vi "VT100Codes.vi"(10 "read buffer":string="\u001b[0m\u001b[01;34mmicropython-serial-0.3\u001b[0m         \u001b[01;34mrequests-2.22.0\u001b[0m\n\u001b[01;31mmicropython-serial-0.3.tar.gz\u001b[0m  \u001b[01;31mrequests-2.22.0.tar.gz\u001b[0m\nrobot@ev3dev:~$ ", 11 "Console In":string="\r\n\r\nLinux ev3dev 4.14.117-ev3dev-2.3.4-ev3 #1 PREEMPT Thu May 9 15:13:01 CDT 2019 armv5tejl\r\n             _____     _\r\n   _____   _|___ /  __| | _____   __\r\n  / _ \\ \\ / / |_ \\ / _` |/ _ \\ \\ / /\r\n |  __/\\ V / ___) | (_| |  __/\\ V /\r\n  \\___| \\_/ |____/ \\__,_|\\___| \\_/\r\n\r\nDebian stretch on LEGO MINDSTORMS EV3!\r\nLast login: Thu Feb 13 18:25:48 2020 from 130.64.189.217\r\r\nrobot@ev3dev:~$ \r\nrobot@ev3dev:~$ \r\nrobot@ev3dev:~$ brickrun -r --  pybricks-micropython\r\nPybricks MicroPython fc828f94 on 2020-01-30; linux version\r\nUse Ctrl-D to exit, Ctrl-E for paste mode\r\n>>> \nrobot@ev3dev:~$ ls\n") -> (3 "Console Out":string="\r\n\r\nLinux ev3dev 4.14.117-ev3dev-2.3.4-ev3 #1 PREEMPT Thu May 9 15:13:01 CDT 2019 armv5tejl\r\n             _____     _\r\n   _____   _|___ /  __| | _____   __\r\n  / _ \\ \\ / / |_ \\ / _` |/ _ \\ \\ / /\r\n |  __/\\ V / ___) | (_| |  __/\\ V /\r\n  \\___| \\_/ |____/ \\__,_|\\___| \\_/\r\n\r\nDebian stretch on LEGO MINDSTORMS EV3!\r\nLast login: Thu Feb 13 18:25:48 2020 from 130.64.189.217\r\r\nrobot@ev3dev:~$ \r\nrobot@ev3dev:~$ \r\nrobot@ev3dev:~$ brickrun -r --  pybricks-micropython\r\nPybricks MicroPython fc828f94 on 2020-01-30; linux version\r\nUse Ctrl-D to exit, Ctrl-E for paste mode\r\n>>> ")   [LabVIEW 2020]
uses:
  ColorText/ColorGlobals.vi
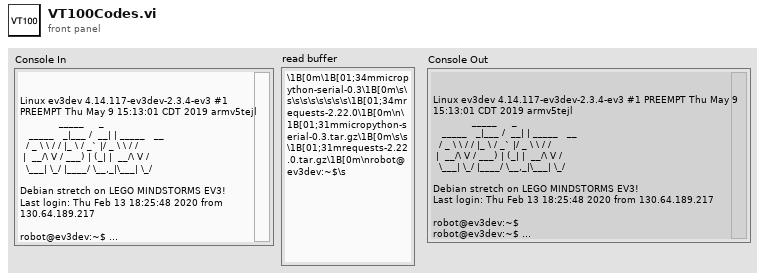
[diagram p1: front panel]
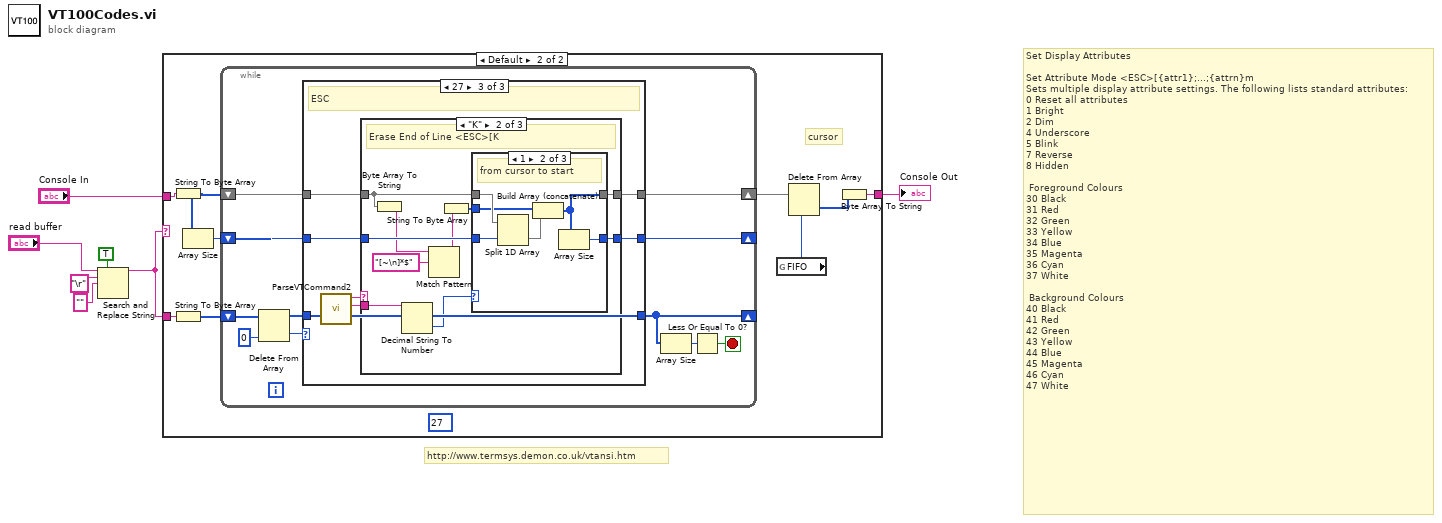
[diagram p0: block diagram]
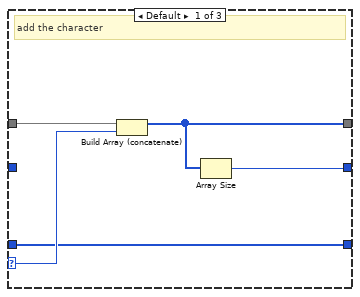
[diagram p3: hidden frame]
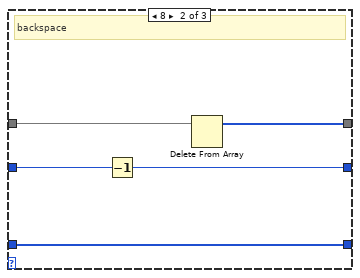
[diagram p4: hidden frame]
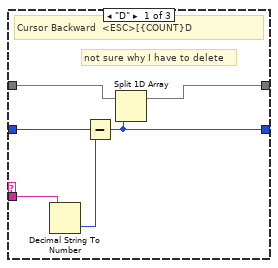
[diagram p5: hidden frame]
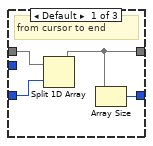
[diagram p6: hidden frame]
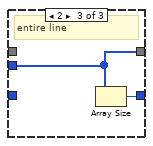
[diagram p7: hidden frame]
diagram:
  # "http://www.termsys.demon.co.uk/vtansi.htm"
  # "Set Display Attributes\n\nSet Attribute Mode\t<ESC>[{attr1};...;{attrn}m\nSets multiple display attribute settings. The following lists standard attributes:\n0\tReset all attributes\n1\tBright\n2\tDim\n4\tUnderscore\t\n5\tBlink\n7\tReverse\n8\tHidden\n\n\tForeground Colours\n30\tBlack\n31\tRed\n32\tGreen\n33\tYellow\n34\tBlue\n35\tMagenta\n36\tCyan\n37\tWhite\n\n\tBackground Colours\n40\tBlack\n41\tRed\n42\tGreen\n43\tYellow\n44\tBlue\n45\tMagenta\n46\tCyan\n47\tWhite"
  n1 = Search and Replace String(replace all?=TRUE ("replace all? (F)"), input string="read buffer", search string="\r" ("replace string (\"\")"), replace string="" ("replace string (\"\")")) -> (result string=w1:string)  [unwired: 4 in, 3 out]
  n2 = case shown="Default" w1 {
    tunnel: "Console In" -> [w8 w14]
    tunnel: w1 -> [_ w13]
    tunnel: [w8 w12] -> w6
    frame "" {
    }
    frame Default {
      (unwired) 27
      # "cursor"
      n3 = String To Byte Array(string=w14) -> (unsigned byte array=w16:u8[])
      n4 = String To Byte Array(string=w13) -> (unsigned byte array=w15:u8[])
      n5 = Array Size(array=w16) -> (size(s)=w17:i32)
      n6 = while {
        shift-right: [w27] -> w11
        shift-left: w16 -> [w28]
        shift-right: [w26] -> _
        shift-left: w17 -> [w25]
        shift-right: [w21] -> _
        shift-left: w15 -> [w24]
        stop <- w19 stop-if-true
        n7 = Delete From Array(array=w24, index=0) -> (deleted portion=w23:u8, array with subset deleted=w22:u8[])  [unwired: 1 in]
        n8 = case shown="27" w23 {
          selector: w23 -> [w32 _ _]
          tunnel: w28 -> [w33 w35 w43]
          tunnel: [w31 w34 w42] -> w27
          tunnel: [w30 w37 w41] -> w26
          tunnel: w25 -> [_ w38 w40]
          tunnel: [w29 w36 w45] -> w21
          tunnel: w22 -> [w29 w36 w46]
          frame Default {
            # "add the character"
            n9 = Build Array (concatenate)(w33, w32) -> (w31:u8[])
            n10 = Array Size(array=w31) -> (size(s)=w30:i32)
          }
          frame 8 {
            # "backspace"
            n11 = Decrement(x=w38) -> (x-1=w37:i32)
            n12 = Delete From Array(array=w35) -> (array with subset deleted=w34:u8[])  [unwired: 2 in, 1 out]
          }
          frame 27 {
            # "ESC"
            n13 = call "ParseVTCommand2.vi"("read buffer"=w46) -> ("VT data"=w39:string, "VT Cmd"=w44:string, "remaining"=w45:u8[])  [unwired: 6 in, 2 out]
            n14 = case shown="\"K\"" w44 {
              tunnel: w43 -> [w49 w57 w76]
              tunnel: [w47 w58 w76] -> w42
              tunnel: [w48 w60 w75] -> w41
              tunnel: w40 -> [w52 w62 w75]
              tunnel: w39 -> [w51 w61 _]
              frame "D" {
                # "not sure why I have to delete"
                # "Cursor Backward\t\t<ESC>[{COUNT}D"
                n15 = Decimal String To Number(string=w51) -> (number=w50:i32)  [unwired: 2 in, 1 out]
                n16 = Subtract(x=w52, y=w50) -> (x-y=w48:i32)
                n17 = Split 1D Array(array=w49, index=w48) -> (first subarray=w47:u8[])  [unwired: 1 out]
              }
              frame "K" {
                # "Erase End of Line\t<ESC>[K"
                n18 = Byte Array To String(unsigned byte array=w57) -> (string=w54:string)
                n19 = Decimal String To Number(string=w61) -> (number=w59:i32)  [unwired: 2 in, 1 out]
                n20 = Match Pattern(string=w54, regular expression="[~\n]*$") -> (before substring=w53:string)  [unwired: 1 in, 3 out]
                n21 = String To Byte Array(string=w53) -> (unsigned byte array=w56:u8[])
                n22 = case shown="1" w59 {
                  tunnel: w62 -> [w65 w71 _]
                  tunnel: [w64 w70 w74] -> w60
                  tunnel: [w63 w67 w73] -> w58
                  tunnel: w57 -> [w66 w72 _]
                  tunnel: w56 -> [_ w69 w73]
                  frame Default {
                    # "from cursor to end"
                    n23 = Split 1D Array(array=w66, index=w65) -> (first subarray=w63:u8[])  [unwired: 1 out]
                    n24 = Array Size(array=w63) -> (size(s)=w64:i32)
                  }
                  frame 1 {
                    # "from cursor to start"
                    n25 = Split 1D Array(array=w72, index=w71) -> (second subarray=w68:u8[])  [unwired: 1 out]
                    n26 = Build Array (concatenate)(w69, w68) -> (w67:u8[])
                    n27 = Array Size(array=w67) -> (size(s)=w70:i32)
                  }
                  frame 2 {
                    # "entire line"
                    n28 = Array Size(array=w73) -> (size(s)=w74:i32)
                  }
                }
              }
              frame Default {
              }
            }
          }
        }
        n29 = Array Size(array=w21) -> (size(s)=w20:i32)
        n30 = Less Or Equal To 0?(x=w20) -> (x <= 0?=w19:bool)
      }
      n31 = global read "ColorGlobals.vi" "FIFO"() -> (w9:i32)
      n32 = Delete From Array(array=w11, length=w9) -> (deleted portion=w10:u8[])  [unwired: 1 in, 1 out]
      n33 = Byte Array To String(unsigned byte array=w10) -> (string=w12:string)
    }
  }
  "Console Out" <- w6
